vi "AMC e.bloxx Query.vi"(8 "error in (no error)":errorcluster, 9 "Module Command":string, 10 "Module Address":i32, 11 "VISA Resource Name":refnum<visa-resource-name>) -> (0 "error out":errorcluster, 1 "Module Response":string, 3 "VISA Resource Name out":refnum<visa-resource-name>)   [LabVIEW 2016]
doc: "<B>AMC - Analytik & Messtechnik GmbH Chemnitz</B>\n\nLabVIEW Drivers for e.bloxx series from Gantner Instruments\n\nThis VI is a driver subroutine and should not be used in an application. It assembles a module command string out of the parameters and writes it to the serial interface specified in <B>VISA Resource Name</B>. Followed by the module command the response is read from the serial interface and provided in <B>Module Response</B>."
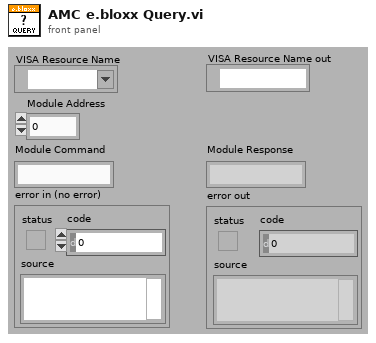
[diagram p1: front panel]
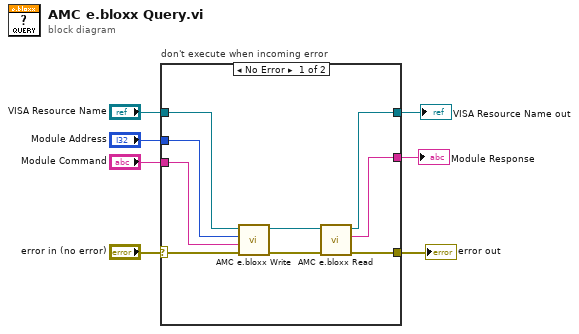
[diagram p0: block diagram]
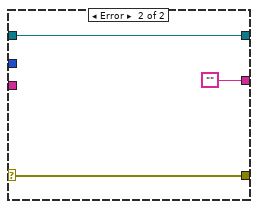
[diagram p2: hidden frame]
diagram:
  n1 = case "don't execute when incoming error" shown="No Error" "error in (no error)" {
    selector: "error in (no error)" -> [w16 w19]
    tunnel: [w9 w19] -> w6
    tunnel: "VISA Resource Name" -> [w13 w18]
    tunnel: "Module Command" -> [w15 _]
    tunnel: "Module Address" -> [w14 _]
    tunnel: [w10 ""] -> w2
    tunnel: [w8 w18] -> w1
    frame No Error {
      n2 = call "AMC e.bloxx Write.vi"("error in (no error)"=w16, "Module Command"=w15, "Module Address"=w14, "VISA Resource Name"=w13) -> ("error out"=w11:errorcluster, "VISA Resource Name out"=w12:refnum<visa-resource-name>)  [unwired: 6 in]
      n3 = call "AMC e.bloxx Read.vi"("error in (no error)"=w11, "VISA Resource Name"=w12) -> ("error out"=w9:errorcluster, "Module Response"=w10:string, "VISA Resource Name out"=w8:refnum<visa-resource-name>)  [unwired: 7 in]
    }
    frame Error {
    }
  }
  "error out" <- w6
  "VISA Resource Name out" <- w1
  "Module Response" <- w2
